vi "createGraph.vi"(7 "robotPos":cluster{"xPos":dbl, "yPos":dbl, "theta":dbl}, 8 "error in":errorcluster caption="error in (no error)", 10 "Direction":dbl[](array[numeric]), 11 "Magnitude":dbl[](array[numeric])) -> (0 "error out":errorcluster, 3 "line out":cluster{"Line":cluster{"X":dbl, "Y":dbl}[]}[](array[cluster]))   [LabVIEW 2016]
uses:
  <vilib>/Analysis/coordinate.llb/Angle Range (Degree).ctl
  <vilib>/Analysis/coordinate.llb/Angle Units.ctl
  <vilib>/Analysis/coordinate.llb/Wrap Angle (scalar).vi
  <vilib>/Analysis/NI_AAL_Angle.lvlib
panel:
  in  "minDist":dbl=100.0
  out "XY Graph":cluster{"Y":dbl[], "Y":dbl[]}[](graph)
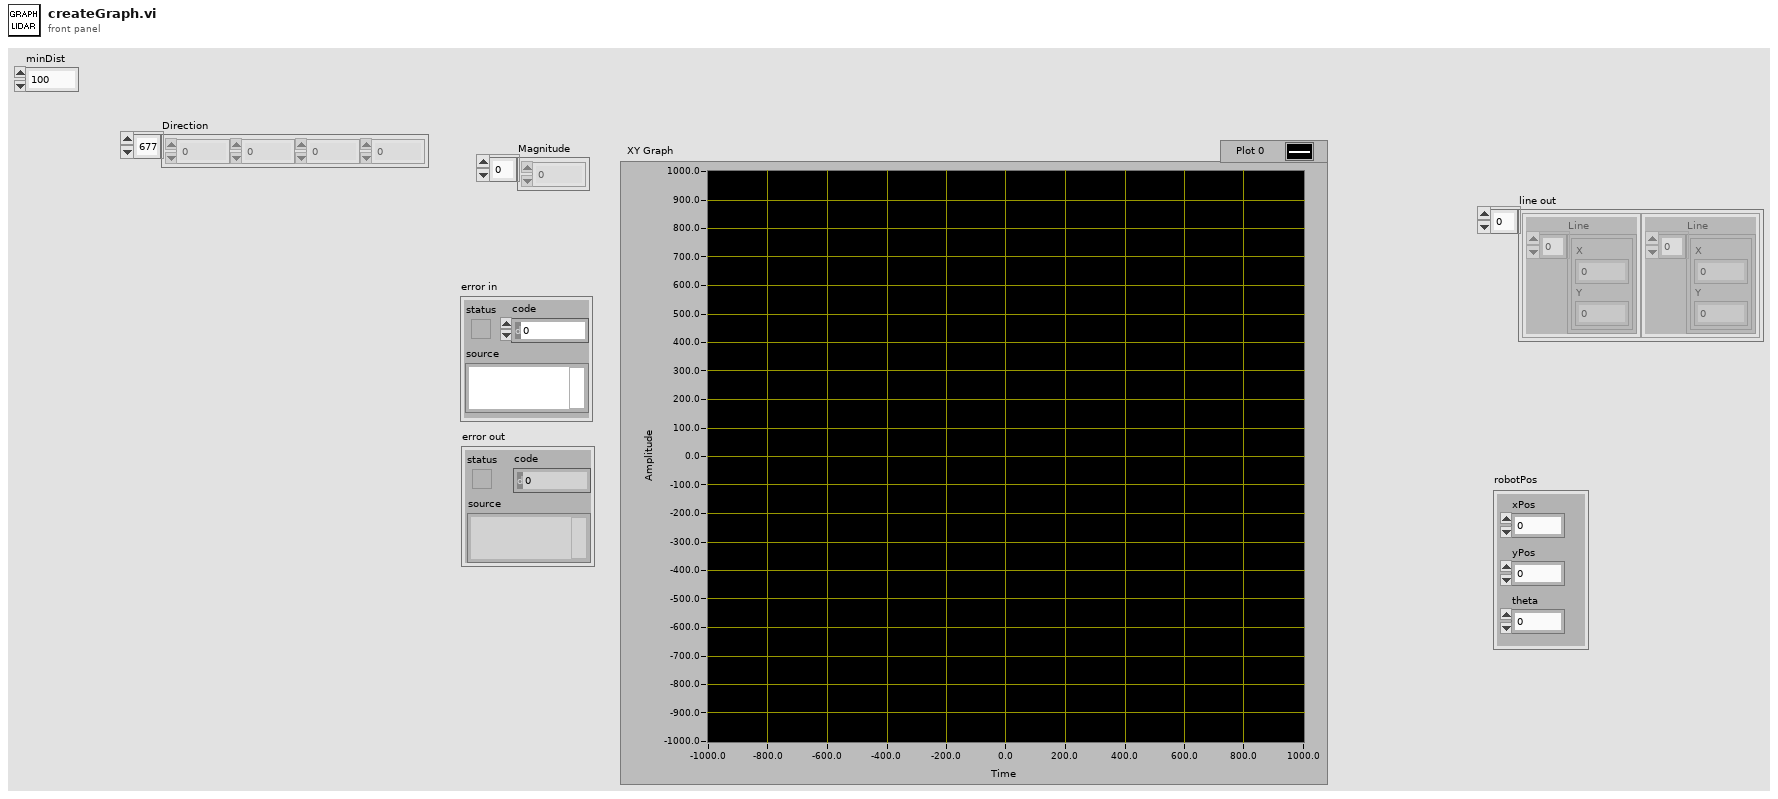
[diagram p1: front panel]
types:
  T1 = typedef "NI_AAL_Angle.lvlib/Angle Units.ctl" = i32
  T2 = typedef "NI_AAL_Angle.lvlib/Angle Range (Degree).ctl" = u16
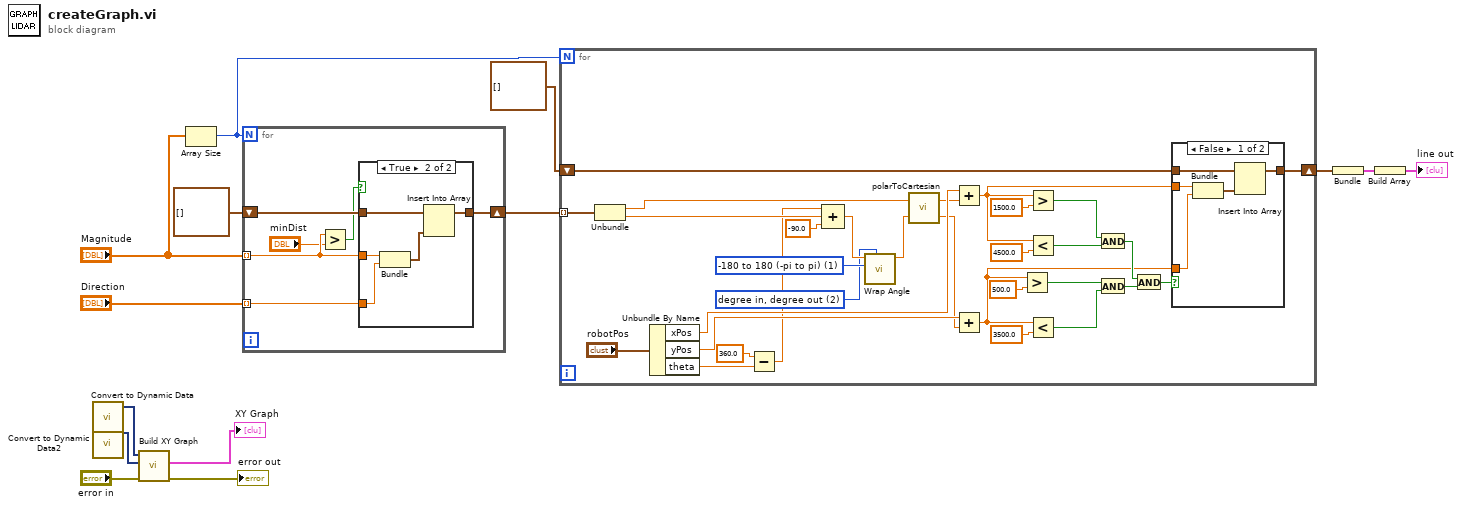
[diagram p0: block diagram]
diagram:
  n1 = call "Convert to Dynamic Data"() -> ("Dynamic Data Type"=w13:dynamicdata)  [unwired: 4 in]
  n2 = call "Convert to Dynamic Data2"() -> ("Dynamic Data Type"=w14:dynamicdata)  [unwired: 4 in]
  n3 = call "Build XY Graph"("error in (no error)"="error in", "Y Input"=w14, "X Input"=w13) -> ("error out"=→"error out":errorcluster, "XY Graph"=→"XY Graph":cluster{"X":dbl[], "Y":dbl[]}[])  [unwired: 7 in]
  n4 = Array Size(array="Magnitude") -> (size(s)=w11:i32)
  n5 = for {
    N: w11 -> [_]
    shift-right: [w18] -> w10
    shift-left: cluster{dbl, dbl}[] [] -> [w19]
    tunnel: "Magnitude" -> [w16] mode=indexing
    tunnel: "Direction" -> [w20] mode=indexing
    n6 = Greater?(x=w16, y="minDist") -> (0:w17:bool)
    n7 = case shown="True" w17 {
      tunnel: w16 -> [_ w26]
      tunnel: w20 -> [_ w25]
      tunnel: w19 -> [w21 w24]
      tunnel: [w21 w23] -> w18
      frame False {
      }
      frame True {
        n8 = Bundle(w26, w25) -> (w22:cluster{dbl, dbl})  [unwired: 1 in]
        n9 = Insert Into Array(array=w24, new element=w22) -> (w23:cluster{dbl, dbl}[])  [unwired: 1 in]
      }
    }
  }
  n10 = for {
    N: w11 -> [_]
    tunnel: w10 -> [w57] mode=indexing
    shift-right: [w27] -> w3
    shift-left: cluster{dbl, dbl}[] [] -> [w55]
    w44 = T1 2 items=["radian in, radian out", "radian in, degree out", "degree in, degree out", "degree in, radian out"] ("angle units")
    w45 = T2 1 items=["none", "-180 to 180 (-pi to pi)", "0 to 360 (0 to 2pi)"] ("angle range")
    n11 = Unbundle(w57) -> (w56:dbl, w49:dbl)
    n12 = Unbundle By Name("robotPos") -> ("xPos"=w53:dbl, "yPos"=w51:dbl, "theta"=w30:dbl)
    n13 = Subtract(x=360.0, y=w30) -> (x-y=w28:dbl)
    n14 = Compound Arithmetic op=ADD(w28, w49, -90.0 ("value")) -> (w47:dbl)
    n15 = call-poly <vilib>:"Wrap Angle.vi"("angle units"=w44, "angle range"=w45, "angle in"=w47) -> ("angle out"=w46:dbl)  [unwired: 7 in, 1 out]
    n16 = call "polarToCartesian.vi"("Angle (deg)"=w46, "Magnitude (r)"=w56) -> ("y"=w50:dbl, "x"=w52:dbl)
    n17 = Add(x=w53, y=w52) -> (x+y=w37:dbl)
    n18 = Add(x=w51, y=w50) -> (x+y=w32:dbl)
    n19 = Greater?(x=w32, y=500.0) -> (0:w41:bool)
    n20 = Greater?(x=w37, y=1500.0) -> (0:w43:bool)
    n21 = Less?(x=w37, y=4500.0) -> (x < y?=w42:bool)
    n22 = Less?(x=w32, y=3500.0) -> (x < y?=w40:bool)
    n23 = And(x=w43, y=w42) -> (x .and. y?=w38:bool)
    n24 = And(x=w41, y=w40) -> (x .and. y?=w39:bool)
    n25 = And(x=w38, y=w39) -> (x .and. y?=w31:bool)
    n26 = case shown="False" w31 {
      tunnel: [w62 w63] -> w27
      tunnel: w55 -> [w58 w63]
      tunnel: w37 -> [w60 _]
      tunnel: w32 -> [w59 _]
      frame False {
        n27 = Bundle(w60, w59) -> (w61:cluster{dbl, dbl})  [unwired: 1 in]
        n28 = Insert Into Array(array=w58, new element=w61) -> (w62:cluster{dbl, dbl}[])  [unwired: 1 in]
      }
      frame True {
      }
    }
  }
  n29 = Bundle(w3) -> (w2:cluster{cluster{dbl, dbl}[]})  [unwired: 1 in]
  n30 = Build Array(w2) -> (→"line out":cluster{cluster{dbl, dbl}[]}[])
